vi "Input Check_TBL.vi"(8 "에러 입력":errorcluster caption="에러 입력(에러 없음)", 11 "Table 참조":refnum<vi>) -> (0 "에러 출력":errorcluster, 1 "Caption.Text":string, 2 "내용있음?":bool, 3 "참조 출력":refnum<vi>)   [LabVIEW 2020]
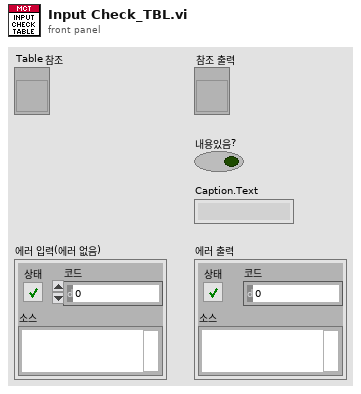
[diagram p1: front panel]
types:
  T1 = enum8{"Enabled", "Disabled", "Disabled and Grayed Out"}
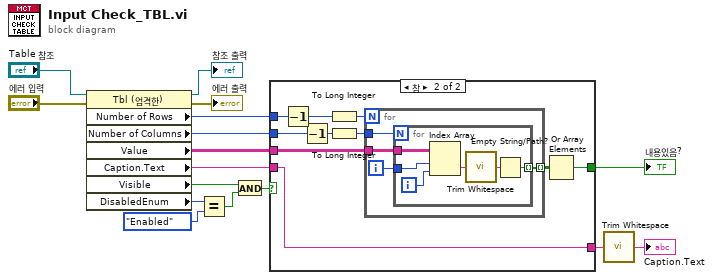
[diagram p0: block diagram]
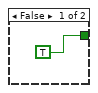
[diagram p2: hidden frame]
diagram:
  n1 = property class="Tbl (엄격한)"(reference="Table 참조", error in="에러 입력") -> (reference out=→"참조 출력":refnum<vi>, error out=→"에러 출력":errorcluster, "Number of Rows"=w14:u32, "Number of Columns"=w13:u32, "Value"=w11:string[][], "Caption.Text"=w10:string, "Visible"=w3:bool, "DisabledEnum"=w5:T1)
  n2 = Equal?(x=w5, y=T1."Enabled" ("비활성화")) -> (x = y?=w2:bool)
  n3 = And(x=w3, y=w2) -> (x .and. y?=w1:bool)
  n4 = case shown="참" w1 {
    tunnel: [TRUE w27] -> w16
    tunnel: w14 -> [_ w21]
    tunnel: w13 -> [_ w20]
    tunnel: w11 -> [_ w19]
    tunnel: w10 -> [_ w18]
    tunnel: [_ w18] -> w8
    frame False {
    }
    frame True {
      n5 = Decrement(x=w21) -> (x-1=w22:u32)
      n6 = Decrement(x=w20) -> (x-1=w23:u32)
      n7 = To Long Integer(number=w22) -> (32bit integer=w25:i32)
      n8 = To Long Integer(number=w23) -> (32bit integer=w24:i32)
      n9 = for {
        N: w25 -> [_]
        tunnel: w19 -> [w30]
        tunnel: w24 -> [w31]
        tunnel: [w29] -> w26 mode=indexing
        i -> [w28]
        n10 = for {
          N: w31 -> [_]
          tunnel: w30 -> [w35]
          tunnel: [w36] -> w29 mode=indexing
          tunnel: w28 -> [w33]
          i -> [w32]
          n11 = Index Array(array=w35, index (row)=w33, index (col)=w32) -> (element=w34:string)
          n12 = call <vilib>:"Trim Whitespace.vi"("string"=w34) -> ("trimmed string"=w37:string)  [unwired: 1 in]
          n13 = Empty String/Path?(string/path=w37) -> (empty?=w36:bool)
        }
      }
      n14 = Or Array Elements(Boolean array=w26) -> (logical OR=w27:bool)
    }
  }
  "내용있음?" <- w16
  n15 = call <vilib>:"Trim Whitespace.vi"("string"=w8) -> ("trimmed string"=→"Caption.Text":string)  [unwired: 1 in]
